vi "CurrentCorrection.vi"(1 "Action":T1(ring), 3 "Current IN":dbl[](array[numeric]), 4 "settling\ndelay":i32) -> (5 "Current OUT":dbl[](array[numeric]), 6 "ProbeStationControl out":refnum<class "ProbeStationControl.lvclass">, 7 "Compliance exceeded?":bool, 8 "Current Reference 100V":dbl[](array[numeric]), 9 "Current Reference 10V":dbl[](array[numeric]))   [LabVIEW 2013]
uses:
  InstrControl/ProbeStationControl/ProbeStationControl.lvclass
  InstrControl/Switching/Switching.lvclass
  general_VIs/globals/QC_MeasurementSetup.vi
  InstrControl/SupplyControl/SupplyControl.lvclass
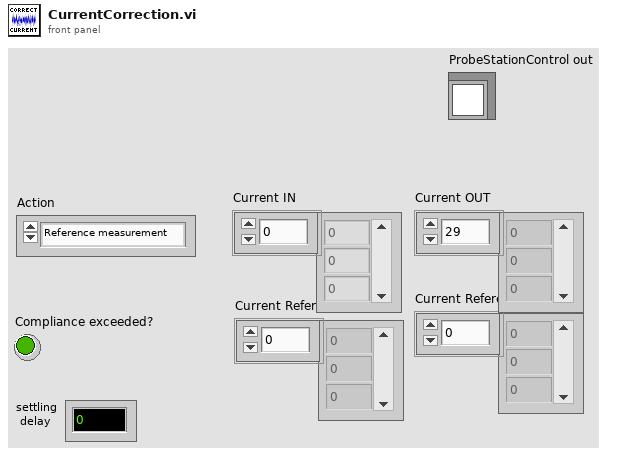
[diagram p1: front panel]
types:
  T1 = enum16{"Reference measurement", "Baseline correcetion 10V", "Baseline correcetion 100V", "Nothing"}
  T2 = cluster{"Bias Supply":refnum<class "SupplyControl.lvclass">, "SMU":refnum<class "SupplyControl.lvclass">, "LCR":refnum<class "LCRControl.lvclass">, "ProbeStation":refnum<class "ProbeStationControl.lvclass">, "Arduino":refnum<class "ArduinoControl.lvclass">, "Measurement switch":refnum<class "Switching.lvclass">, "Probe Card Channels":i32, "Bias Voltage [V]":dbl, "First strip":i32, "Last strip":i32, "Base Voltage [V]":dbl, "Base Ramp Step [V]":dbl, "Base Ramp Interval [ms]":u32, "High Voltage [V]":dbl, "High Ramp Step [V]":dbl, "High Ramp Interval [ms]":u32, "AC frequency [Hz]":i32, "AC amplitude [V]":dbl, "RC Configuration":u16, "Single Needle":bool, "Temperature Readout":enum16{"Read Arduino", "Enter manually"}, "Fraction of good strips [%]":dbl, "Measurement switch used?":bool, "Matrix X Channels":cluster{"Mux1 C1":i32, "Mux1 C2":i32, "Mux2 C1":i32, "Mux2 C2":i32}, "Pinholes Y/N":bool, "Capacitance Y/N":bool, "Resistance Y/N":bool, "Bias Supply Name":string, "SMU Name":string, "LCR Name":string}
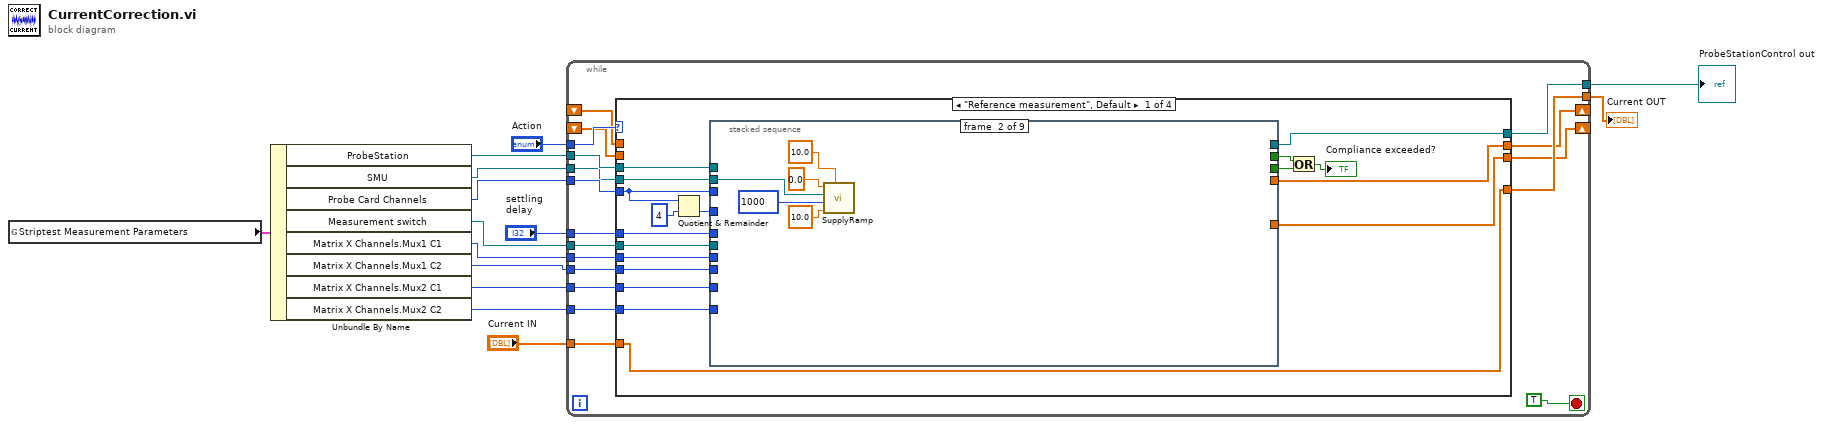
[diagram p0: block diagram]
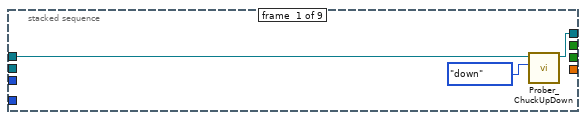
[diagram p2: hidden frame]
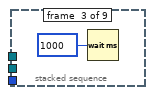
[diagram p3: hidden frame]
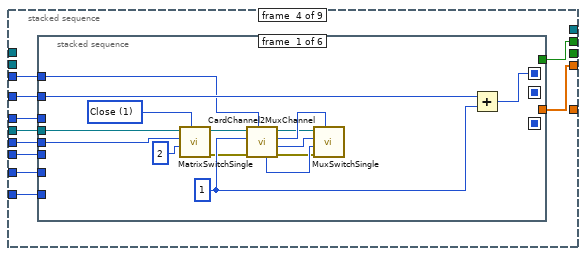
[diagram p4: hidden frame]
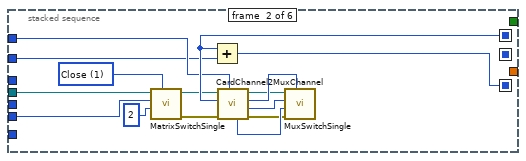
[diagram p5: hidden frame]
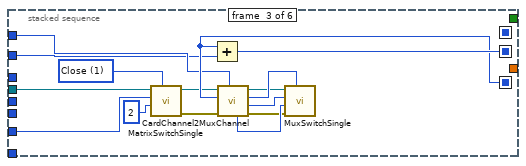
[diagram p6: hidden frame]
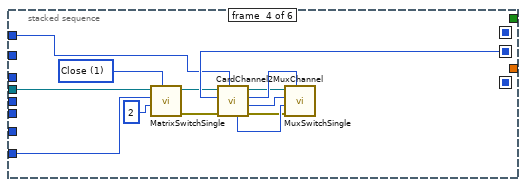
[diagram p7: hidden frame]
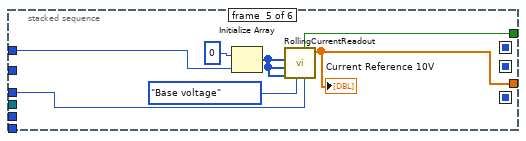
[diagram p8: hidden frame]
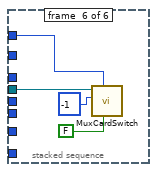
[diagram p9: hidden frame]
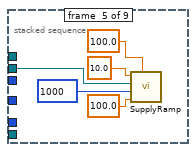
[diagram p10: hidden frame]
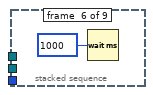
[diagram p11: hidden frame]
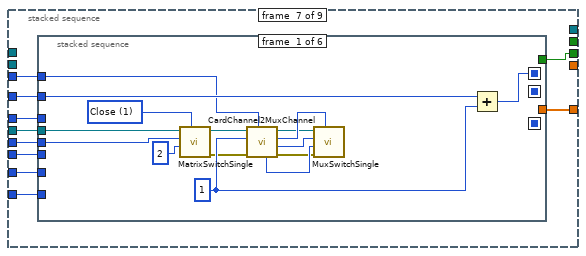
[diagram p12: hidden frame]
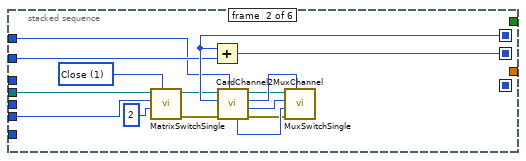
[diagram p13: hidden frame]
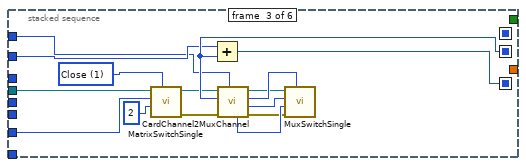
[diagram p14: hidden frame]
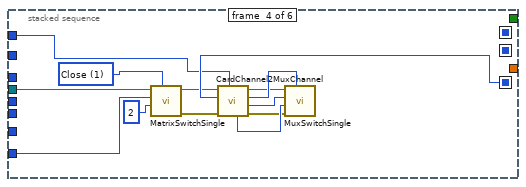
[diagram p15: hidden frame]
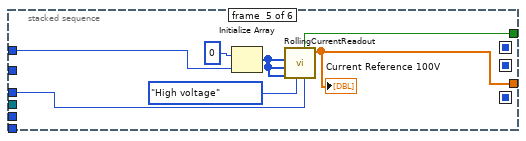
[diagram p16: hidden frame]
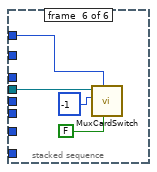
[diagram p17: hidden frame]
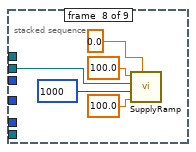
[diagram p18: hidden frame]
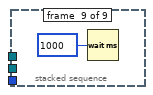
[diagram p19: hidden frame]
diagram:
  n1 = global read "QC_MeasurementSetup.vi" "Striptest Measurement Parameters"() -> (w9:T2)
  n2 = Unbundle By Name(w9) -> ("ProbeStation"=w1:refnum<class "ProbeStationControl.lvclass">, "SMU"=w8:refnum<class "SupplyControl.lvclass">, "Probe Card Channels"=w7:i32, "Measurement switch"=w6:refnum<class "Switching.lvclass">, "Matrix X Channels.Mux1 C1"=w5:i32, "Matrix X Channels.Mux1 C2"=w4:i32, "Matrix X Channels.Mux2 C1"=w3:i32, "Matrix X Channels.Mux2 C2"=w2:i32)
  n3 = while {
    tunnel: "Action" -> [w32]
    tunnel: w7 -> [w31]
    tunnel: [w30] -> w13
    tunnel: "Current IN" -> [w29]
    shift-right: [w27] -> _
    shift-left: _ -> [w25]
    shift-right: [w26] -> _
    shift-left: _ -> [w24]
    tunnel: "settling\ndelay" -> [w23]
    tunnel: w1 -> [w22]
    tunnel: [w21] -> w10
    tunnel: w8 -> [w20]
    tunnel: w6 -> [w19]
    tunnel: w5 -> [w18]
    tunnel: w4 -> [w17]
    tunnel: w3 -> [w16]
    tunnel: w2 -> [w15]
    stop <- TRUE stop-if-true
    n4 = case shown="\"Reference measurement\", Default" w32 {
      tunnel: w31 -> [w39 _ w239 w247]
      tunnel: [w50 w233 w238 w246] -> w30
      tunnel: w29 -> [w50 w233 w237 w248]
      tunnel: [w46 w231 w236 w244] -> w27
      tunnel: [w45 w232 w235 w245] -> w26
      tunnel: w25 -> [_ w231 w236 w244]
      tunnel: w24 -> [_ w232 w235 w245]
      tunnel: w23 -> [w44 _ _ _]
      tunnel: w22 -> [w43 w230 w234 w243]
      tunnel: [w42 w230 w234 w243] -> w21
      tunnel: w20 -> [w41 _ _ _]
      tunnel: w19 -> [w37 _ _ _]
      tunnel: w18 -> [w36 _ _ _]
      tunnel: w17 -> [w35 _ _ _]
      tunnel: w16 -> [w34 _ _ _]
      tunnel: w15 -> [w33 _ _ _]
      frame "Reference measurement", Default {
        n5 = Quotient & Remainder(x=w39, y=4) -> (floor(x/y)=w38:i32)  [unwired: 1 out]
        n6 = stacked-sequence {
          tunnel: w39 -> [_ _ _ w64 _ _ w150 _ _]
          tunnel: [_ _ _ w69 _ _ _ _ _] -> w48
          tunnel: [_ _ _ _ _ _ w154 _ _] -> w47
          tunnel: [_ _ _ w68 _ _ _ _ _] -> w46
          tunnel: [_ _ _ _ _ _ w153 _ _] -> w45
          tunnel: w44 -> [_ _ _ w65 _ _ w148 _ _]
          tunnel: w41 -> [_ w54 _ _ w139 _ _ w224 _]
          tunnel: w37 -> [_ _ _ w67 _ _ w152 _ _]
          tunnel: w43 -> [w52 _ _ _ _ _ _ _ _]
          tunnel: [w51 _ _ _ _ _ _ _ _] -> w42
          tunnel: w36 -> [_ _ _ w66 _ _ w151 _ _]
          tunnel: w35 -> [_ _ _ w60 _ _ w145 _ _]
          tunnel: w34 -> [_ _ _ w62 _ _ w146 _ _]
          tunnel: w33 -> [_ _ _ w61 _ _ w147 _ _]
          tunnel: w38 -> [_ _ _ w63 _ _ w149 _ _]
          frame #0 {
            n7 = call-dynamic "Prober_ChuckUpDown.vi"("Direction"=enum16{"up", "down"}."down", "ProbeStationControl in"=w52) -> ("ProbeStationControl out"=w51:refnum<class "ProbeStationControl.lvclass">)  [unwired: 7 in, 2 out]
          }
          frame #1 {
            n8 = call "SupplyRamp.vi"("Requested Voltage"=10.0, "Step Size"=10.0, "Step Delay"=1000, "Supply IN"=w54, "Starting Voltage"=0.0) -> ()  [unwired: 3 in, 4 out]
          }
          frame #2 {
            n9 = Wait (ms)(milliseconds to wait=1000) -> ()  [unwired: 1 out]
          }
          frame #3 {
            n10 = stacked-sequence {
              seq-local: [w75 _ _ _ _ _] -> [_ w94 _ _ _ _]
              seq-local: [_ w93 _ _ _ _] -> [_ _ w108 _ _ _]
              seq-local: [_ _ w109 _ _ _] -> [_ _ _ w122 _ _]
              tunnel: w67 -> [w80 w87 w102 w116 _ w137]
              tunnel: w66 -> [w79 _ _ _ _ _]
              tunnel: w63 -> [w76 w85 w100 _ _ _]
              tunnel: w60 -> [_ w92 _ _ _ _]
              tunnel: w62 -> [_ _ w107 _ _ _]
              tunnel: w61 -> [_ _ _ w121 _ _]
              tunnel: w65 -> [_ _ _ _ w131 _]
              tunnel: w64 -> [w70 w86 w101 w115 w130 w136]
              tunnel: [_ _ _ _ w129 _] -> w69
              tunnel: [_ _ _ _ w128 _] -> w68
              frame #0 {
                w77 = 1
                w78 = u16 1 items=["Open", "Close"] ("Switch action")
                n11 = call-dynamic "MatrixSwitchSingle.vi"("Switch action"=w78, "Matrix Y"=2, "Matrix X"=w79, "Switching in"=w80) -> ("error out"=w72:errorcluster, "Switching out"=w73:refnum<class "Switching.lvclass">)  [unwired: 5 in, 1 out]
                n12 = call-dynamic "CardChannel2MuxChannel.vi"("Probe Card Channels"=w70, "error in (no error)"=w72, "Probecard Channel No."=w77, "Switching in"=w73) -> ("error out"=w71:errorcluster, "C1 / C2"=w83:i32, "Mux No.:"=w82:u32, "Switching out"=w74:refnum<class "Switching.lvclass">, "Channel"=w84:i32)  [unwired: 2 in, 1 out]
                n13 = call-dynamic "MuxSwitchSingle.vi"("MUX address"=w82, "error in (no error)"=w71, "Channel"=w84, "C1 / C2"=w83, "Switching in"=w74) -> ()  [unwired: 4 in, 3 out]
                n14 = Add(x=w76, y=w77) -> (x+y=w75:i32)
              }
              frame #1 {
                w96 = u16 1 items=["Open", "Close"] ("Switch action")
                n15 = call-dynamic "MatrixSwitchSingle.vi"("Switch action"=w96, "Matrix Y"=2, "Matrix X"=w92, "Switching in"=w87) -> ("error out"=w89:errorcluster, "Switching out"=w88:refnum<class "Switching.lvclass">)  [unwired: 5 in, 1 out]
                n16 = Add(x=w94, y=w85) -> (x+y=w93:i32)
                n17 = call-dynamic "CardChannel2MuxChannel.vi"("Probe Card Channels"=w86, "error in (no error)"=w89, "Probecard Channel No."=w94, "Switching in"=w88) -> ("error out"=w91:errorcluster, "C1 / C2"=w98:i32, "Mux No.:"=w97:u32, "Switching out"=w90:refnum<class "Switching.lvclass">, "Channel"=w99:i32)  [unwired: 2 in, 1 out]
                n18 = call-dynamic "MuxSwitchSingle.vi"("MUX address"=w97, "error in (no error)"=w91, "Channel"=w99, "C1 / C2"=w98, "Switching in"=w90) -> ()  [unwired: 4 in, 3 out]
              }
              frame #2 {
                w113 = u16 1 items=["Open", "Close"] ("Switch action")
                n19 = call-dynamic "MatrixSwitchSingle.vi"("Switch action"=w113, "Matrix Y"=2, "Matrix X"=w107, "Switching in"=w102) -> ("error out"=w103:errorcluster, "Switching out"=w104:refnum<class "Switching.lvclass">)  [unwired: 5 in, 1 out]
                n20 = Add(x=w108, y=w100) -> (x+y=w109:i32)
                n21 = call-dynamic "CardChannel2MuxChannel.vi"("Probe Card Channels"=w101, "error in (no error)"=w103, "Probecard Channel No."=w108, "Switching in"=w104) -> ("error out"=w106:errorcluster, "C1 / C2"=w111:i32, "Mux No.:"=w112:u32, "Switching out"=w105:refnum<class "Switching.lvclass">, "Channel"=w110:i32)  [unwired: 2 in, 1 out]
                n22 = call-dynamic "MuxSwitchSingle.vi"("MUX address"=w112, "error in (no error)"=w106, "Channel"=w110, "C1 / C2"=w111, "Switching in"=w105) -> ()  [unwired: 4 in, 3 out]
              }
              frame #3 {
                w124 = u16 1 items=["Open", "Close"] ("Switch action")
                n23 = call-dynamic "MatrixSwitchSingle.vi"("Switch action"=w124, "Matrix Y"=2, "Matrix X"=w121, "Switching in"=w116) -> ("error out"=w117:errorcluster, "Switching out"=w120:refnum<class "Switching.lvclass">)  [unwired: 5 in, 1 out]
                n24 = call-dynamic "CardChannel2MuxChannel.vi"("Probe Card Channels"=w115, "error in (no error)"=w117, "Probecard Channel No."=w122, "Switching in"=w120) -> ("error out"=w118:errorcluster, "C1 / C2"=w126:i32, "Mux No.:"=w125:u32, "Switching out"=w119:refnum<class "Switching.lvclass">, "Channel"=w127:i32)  [unwired: 2 in, 1 out]
                n25 = call-dynamic "MuxSwitchSingle.vi"("MUX address"=w125, "error in (no error)"=w118, "Channel"=w127, "C1 / C2"=w126, "Switching in"=w119) -> ()  [unwired: 4 in, 3 out]
              }
              frame #4 {
                n26 = Initialize Array(0, w130) -> (w134:i32[])
                n27 = call "RollingCurrentReadout.vi"("settling\ndelay"=w131, "Base/High Voltage?"=enum16{"Base voltage", "High voltage"}."Base voltage", "disabled channels IN"=w134, "Flag IN"=w134, "Current Array IN [nA]"=w134) -> ("Current Array OUT [nA]"=w128:dbl[], "Compliance exceeded"=w129:bool)  [unwired: 3 in, 2 out]
                "Current Reference 10V" <- w128
              }
              frame #5 {
                n28 = call-dynamic "MuxCardSwitch.vi"("Single Needle"=FALSE, "Probe Card Channels"=w136, "Switch to channel"=-1, "Switching in"=w137) -> ()  [unwired: 5 in, 3 out]
              }
            }
          }
          frame #4 {
            n29 = call "SupplyRamp.vi"("Requested Voltage"=100.0, "Step Size"=100.0, "Step Delay"=1000, "Supply IN"=w139, "Starting Voltage"=10.0) -> ()  [unwired: 3 in, 4 out]
          }
          frame #5 {
            n30 = Wait (ms)(milliseconds to wait=1000) -> ()  [unwired: 1 out]
          }
          frame #6 {
            n31 = stacked-sequence {
              seq-local: [w160 _ _ _ _ _] -> [_ w179 _ _ _ _]
              seq-local: [_ w178 _ _ _ _] -> [_ _ w194 _ _ _]
              seq-local: [_ _ w193 _ _ _] -> [_ _ _ w207 _ _]
              tunnel: w152 -> [w164 w171 w185 w201 _ w222]
              tunnel: w151 -> [w163 _ _ _ _ _]
              tunnel: w149 -> [w161 w172 w187 _ _ _]
              tunnel: w145 -> [_ w177 _ _ _ _]
              tunnel: w146 -> [_ _ w192 _ _ _]
              tunnel: w147 -> [_ _ _ w206 _ _]
              tunnel: w150 -> [w155 w170 w186 w200 w216 w221]
              tunnel: w148 -> [_ _ _ _ w215 _]
              tunnel: [_ _ _ _ w214 _] -> w154
              tunnel: [_ _ _ _ w213 _] -> w153
              frame #0 {
                w162 = 1
                w169 = u16 1 items=["Open", "Close"] ("Switch action")
                n32 = call-dynamic "MatrixSwitchSingle.vi"("Switch action"=w169, "Matrix Y"=2, "Matrix X"=w163, "Switching in"=w164) -> ("error out"=w159:errorcluster, "Switching out"=w157:refnum<class "Switching.lvclass">)  [unwired: 5 in, 1 out]
                n33 = call-dynamic "CardChannel2MuxChannel.vi"("Probe Card Channels"=w155, "error in (no error)"=w159, "Probecard Channel No."=w162, "Switching in"=w157) -> ("error out"=w158:errorcluster, "C1 / C2"=w167:i32, "Mux No.:"=w166:u32, "Switching out"=w156:refnum<class "Switching.lvclass">, "Channel"=w168:i32)  [unwired: 2 in, 1 out]
                n34 = call-dynamic "MuxSwitchSingle.vi"("MUX address"=w166, "error in (no error)"=w158, "Channel"=w168, "C1 / C2"=w167, "Switching in"=w156) -> ()  [unwired: 4 in, 3 out]
                n35 = Add(x=w161, y=w162) -> (x+y=w160:i32)
              }
              frame #1 {
                w181 = u16 1 items=["Open", "Close"] ("Switch action")
                n36 = call-dynamic "MatrixSwitchSingle.vi"("Switch action"=w181, "Matrix Y"=2, "Matrix X"=w177, "Switching in"=w171) -> ("error out"=w176:errorcluster, "Switching out"=w174:refnum<class "Switching.lvclass">)  [unwired: 5 in, 1 out]
                n37 = Add(x=w179, y=w172) -> (x+y=w178:i32)
                n38 = call-dynamic "CardChannel2MuxChannel.vi"("Probe Card Channels"=w170, "error in (no error)"=w176, "Probecard Channel No."=w179, "Switching in"=w174) -> ("error out"=w175:errorcluster, "C1 / C2"=w183:i32, "Mux No.:"=w182:u32, "Switching out"=w173:refnum<class "Switching.lvclass">, "Channel"=w184:i32)  [unwired: 2 in, 1 out]
                n39 = call-dynamic "MuxSwitchSingle.vi"("MUX address"=w182, "error in (no error)"=w175, "Channel"=w184, "C1 / C2"=w183, "Switching in"=w173) -> ()  [unwired: 4 in, 3 out]
              }
              frame #2 {
                w198 = u16 1 items=["Open", "Close"] ("Switch action")
                n40 = call-dynamic "MatrixSwitchSingle.vi"("Switch action"=w198, "Matrix Y"=2, "Matrix X"=w192, "Switching in"=w185) -> ("error out"=w191:errorcluster, "Switching out"=w188:refnum<class "Switching.lvclass">)  [unwired: 5 in, 1 out]
                n41 = Add(x=w187, y=w194) -> (x+y=w193:i32)
                n42 = call-dynamic "CardChannel2MuxChannel.vi"("Probe Card Channels"=w186, "error in (no error)"=w191, "Probecard Channel No."=w194, "Switching in"=w188) -> ("error out"=w190:errorcluster, "C1 / C2"=w196:i32, "Mux No.:"=w197:u32, "Switching out"=w189:refnum<class "Switching.lvclass">, "Channel"=w195:i32)  [unwired: 2 in, 1 out]
                n43 = call-dynamic "MuxSwitchSingle.vi"("MUX address"=w197, "error in (no error)"=w190, "Channel"=w195, "C1 / C2"=w196, "Switching in"=w189) -> ()  [unwired: 4 in, 3 out]
              }
              frame #3 {
                w209 = u16 1 items=["Open", "Close"] ("Switch action")
                n44 = call-dynamic "MatrixSwitchSingle.vi"("Switch action"=w209, "Matrix Y"=2, "Matrix X"=w206, "Switching in"=w201) -> ("error out"=w205:errorcluster, "Switching out"=w203:refnum<class "Switching.lvclass">)  [unwired: 5 in, 1 out]
                n45 = call-dynamic "CardChannel2MuxChannel.vi"("Probe Card Channels"=w200, "error in (no error)"=w205, "Probecard Channel No."=w207, "Switching in"=w203) -> ("error out"=w204:errorcluster, "C1 / C2"=w211:i32, "Mux No.:"=w210:u32, "Switching out"=w202:refnum<class "Switching.lvclass">, "Channel"=w212:i32)  [unwired: 2 in, 1 out]
                n46 = call-dynamic "MuxSwitchSingle.vi"("MUX address"=w210, "error in (no error)"=w204, "Channel"=w212, "C1 / C2"=w211, "Switching in"=w202) -> ()  [unwired: 4 in, 3 out]
              }
              frame #4 {
                n47 = Initialize Array(0, w216) -> (w219:i32[])
                n48 = call "RollingCurrentReadout.vi"("settling\ndelay"=w215, "Base/High Voltage?"=enum16{"Base voltage", "High voltage"}."High voltage", "disabled channels IN"=w219, "Flag IN"=w219, "Current Array IN [nA]"=w219) -> ("Current Array OUT [nA]"=w213:dbl[], "Compliance exceeded"=w214:bool)  [unwired: 3 in, 2 out]
                "Current Reference 100V" <- w213
              }
              frame #5 {
                n49 = call-dynamic "MuxCardSwitch.vi"("Single Needle"=FALSE, "Probe Card Channels"=w221, "Switch to channel"=-1, "Switching in"=w222) -> ()  [unwired: 5 in, 3 out]
              }
            }
          }
          frame #7 {
            n50 = call "SupplyRamp.vi"("Requested Voltage"=0.0, "Step Size"=100.0, "Step Delay"=1000, "Supply IN"=w224, "Starting Voltage"=100.0) -> ()  [unwired: 3 in, 4 out]
          }
          frame #8 {
            n51 = Wait (ms)(milliseconds to wait=1000) -> ()  [unwired: 1 out]
          }
        }
        n52 = Or(x=w48, y=w47) -> (x .or. y?=→"Compliance exceeded?":bool)
      }
      frame "Nothing" {
      }
      frame "Baseline correcetion 10V" {
        n53 = for {
          N: w239 -> [_]
          tunnel: w236 -> [w241] mode=indexing
          tunnel: w237 -> [w242] mode=indexing
          tunnel: [w240] -> w238 mode=indexing
          n54 = Subtract(x=w242, y=w241) -> (x-y=w240:dbl)
        }
      }
      frame "Baseline correcetion 100V" {
        n55 = for {
          N: w247 -> [_]
          tunnel: w248 -> [w251] mode=indexing
          tunnel: w245 -> [w250] mode=indexing
          tunnel: [w249] -> w246 mode=indexing
          n56 = Subtract(x=w251, y=w250) -> (x-y=w249:dbl)
        }
      }
    }
  }
  "Current OUT" <- w13
  "ProbeStationControl out" <- w10
